vi "writeLogWindow.vi"(4 "Enable":bool, 6 "Play":bool, 8 "error in (no error)":errorcluster, 9 "On":bool, 10 "FPS":dbl=60.0, 11 "Game in":refnum<class "Game.lvclass">) -> (0 "error out":errorcluster, 3 "Game out":refnum<class "Game.lvclass">)   [LabVIEW 2020, in "Game.lvclass"]
uses:
  Game.lvclass
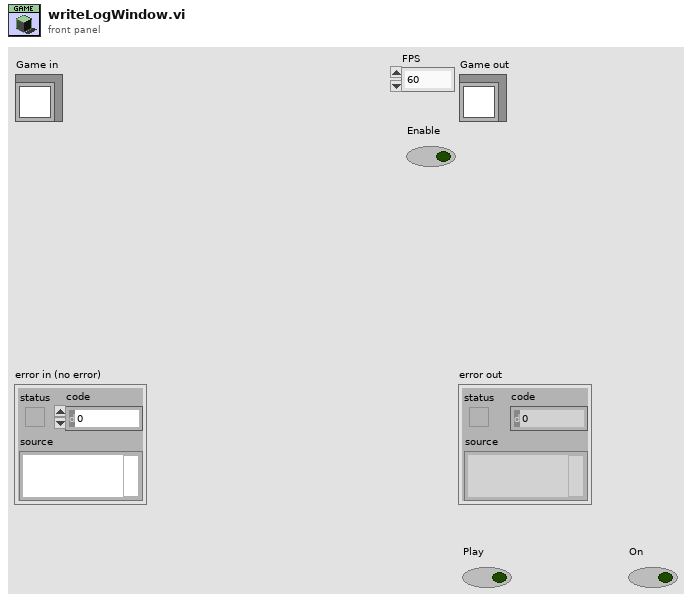
[diagram p1: front panel]
types:
  T1 = enum16{"open", "replace", "create", "open or create", "replace or create", "replace or create with confirmation"}
  T2 = typedef "ReplayInfo.ctl" = cluster{"ByteArrayFromVision":u8[], "TimeStampSampledInReplay":string}
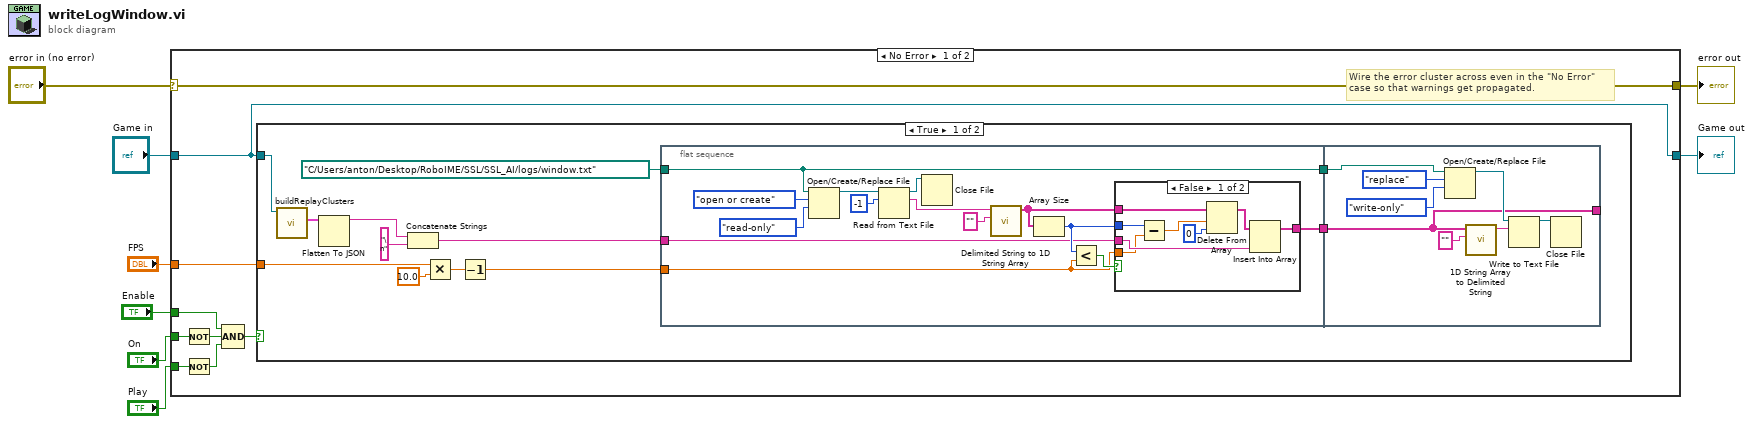
[diagram p0: block diagram]
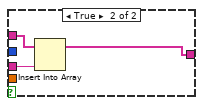
[diagram p2: hidden frame]
diagram:
  n1 = case shown="No Error" "error in (no error)" {
    selector: "error in (no error)" -> [w17 w64]
    tunnel: [w17 w64] -> w7
    tunnel: [w16 w63] -> w5
    tunnel: "Game in" -> [w16 w63]
    tunnel: "FPS" -> [w15 _]
    tunnel: "On" -> [w12 _]
    tunnel: "Play" -> [w14 _]
    tunnel: "Enable" -> [w9 _]
    frame No Error {
      # "Wire the error cluster across even in the \"No Error\"\ncase so that warnings get propagated."
      n2 = Not(x=w12) -> (.not. x?=w11:bool)
      n3 = Not(x=w14) -> (.not. x?=w10:bool)
      n4 = Compound Arithmetic op=AND(w9, w11, w10) -> (w13:bool)
      n5 = case shown="True" w13 {
        tunnel: w16 -> [w29 _]
        tunnel: w15 -> [w25 _]
        frame True {
          n6 = call "buildReplayClusters.vi"("Game in"=w29) -> ("ReplayInfo"=w28:T2)  [unwired: 8 in, 2 out]
          n7 = Flatten To JSON(anything=w28) -> (JSON string=w27:string)  [unwired: 2 in, 1 out]
          n8 = Concatenate Strings(w27, "\n" ("string")) -> (w23:string)
          n9 = Multiply(x=w25, y=10.0) -> (x*y=w22:dbl)
          n10 = Decrement(x=w22) -> (x-1=w21:dbl)
          n11 = flat-sequence {
            tunnel: w23 -> [w36]
            tunnel: w21 -> [w35]
            tunnel: path "C:/Users/anton/Desktop/RoboIME/SSL/SSL_AI/logs/window.txt" ("file (use dialog)") -> [w32]
            tunnel: [w38] -> w19
            tunnel: [w32] -> w18
            tunnel: [w58] -> _
            tunnel: w19 -> [w58]
            tunnel: w18 -> [w57]
            frame #0 {
              n12 = Open/Create/Replace File(file path (use dialog)=w32, operation (0:open)=T1."open or create", access (0:read/write)=enum16{"read/write", "read-only", "write-only"}."read-only") -> (refnum out=w33:refnum<file>)  [unwired: 3 in, 2 out]
              n13 = Read from Text File(file (use dialog)=w33, count=-1) -> (refnum out=w31:refnum<file>, text=w42:string)  [unwired: 2 in, 2 out]
              n14 = Close File(refnum=w31) -> ()  [unwired: 1 in, 2 out]
              n15 = call <vilib>:"Delimited String to 1D String Array.vi"("delimiter"="", "delimited string"=w42) -> ("string array"=w39:string[])  [unwired: 9 in]
              n16 = Array Size(array=w39) -> (size(s)=w37:i32)
              n17 = Less?(x=w37, y=w35) -> (x < y?=w40:bool)
              n18 = case shown="False" w40 {
                tunnel: w39 -> [w51 w54]
                tunnel: w36 -> [w48 w53]
                tunnel: [w47 w52] -> w38
                tunnel: w37 -> [w46 _]
                tunnel: w35 -> [w45 _]
                frame False {
                  n19 = Subtract(x=w46, y=w45) -> (x-y=w44:dbl)
                  n20 = Delete From Array(array=w51, length=w44, index=0) -> (array with subset deleted=w49:string[])  [unwired: 1 out]
                  n21 = Insert Into Array(array=w49, new element=w48) -> (w47:string[])  [unwired: 1 in]
                }
                frame True {
                  n22 = Insert Into Array(array=w54, new element=w53) -> (w52:string[])  [unwired: 1 in]
                }
              }
            }
            frame #1 {
              n23 = Open/Create/Replace File(file path (use dialog)=w57, operation (0:open)=T1."replace", access (0:read/write)=enum16{"read/write", "read-only", "write-only"}."write-only") -> (refnum out=w62:refnum<file>)  [unwired: 3 in, 2 out]
              n24 = call <vilib>:"1D String Array to Delimited String.vi"("delimiter"="", "string array"=w58) -> ("delimited string"=w60:string)  [unwired: 9 in]
              n25 = Write to Text File(file (use dialog)=w62, text=w60) -> (refnum out=w56:refnum<file>)  [unwired: 2 in, 2 out]
              n26 = Close File(refnum=w56) -> ()  [unwired: 1 in, 2 out]
            }
          }
        }
        frame False {
        }
      }
    }
    frame Error {
    }
  }
  "error out" <- w7
  "Game out" <- w5
